vi "Stop Count Down.vi"(8 "error in (no error)":errorcluster, 11 "Work in":refnum<class "Work.lvclass">) -> (0 "error out":errorcluster, 3 "Work out":refnum<class "Work.lvclass">)   [LabVIEW 2024, in "Chef State.lvlib" / "Work.lvclass"]
uses:
  Work.lvclass
  <vilib>/ActorFramework/Message Enqueuer/Message Enqueuer.lvclass/Message Enqueuer.ctl
  Work.lvclass/Work.ctl
  Worker/Worker Messages/Stop Count Down Msg/Stop Count Down Msg.lvclass
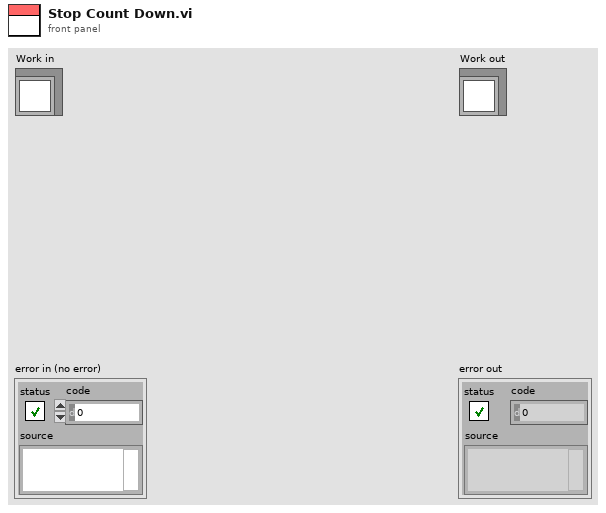
[diagram p1: front panel]
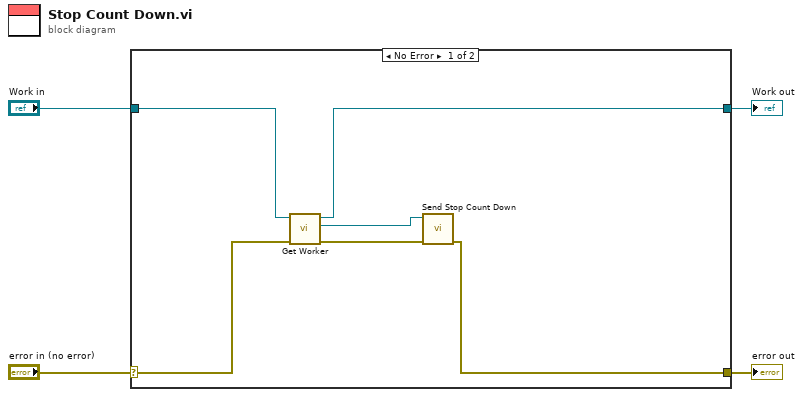
[diagram p0: block diagram]
diagram:
  n1 = case shown="No Error" "error in (no error)" {
    selector: "error in (no error)" -> [w10 w12]
    tunnel: [w6 w12] -> w3
    tunnel: [w8 w11] -> w1
    tunnel: "Work in" -> [w9 w11]
    frame No Error {
      n2 = call-dynamic "Get Worker.vi"("error in (no error)"=w10, "Chef State in"=w9) -> ("error out"=w7:errorcluster, "Worker"=w5:refnum<class "Message Enqueuer.lvclass">, "Chef State out"=w8:refnum<class "Work.lvclass">)  [unwired: 7 in]
      n3 = call "Send Stop Count Down.vi"("error in (no error)"=w7, "Message Enqueuer"=w5) -> ("error out"=w6:errorcluster)  [unwired: 8 in, 1 out]
    }
    frame Error {
    }
  }
  "error out" <- w3
  "Work out" <- w1
